vi "Stop Streaming.vi"(8 "error in (no error)":errorcluster, 11 "Camera in":refnum<class "Camera.lvclass">) -> (0 "error out":errorcluster, 3 "Camera":refnum<class "Camera.lvclass">)   [LabVIEW 2020, in "Camera.lvclass"]
doc: "Stop the camera streaming."
uses:
  Camera.lvclass
  Camera.lvclass/Camera.ctl
  bin/gindustrialcam_32-1.dll
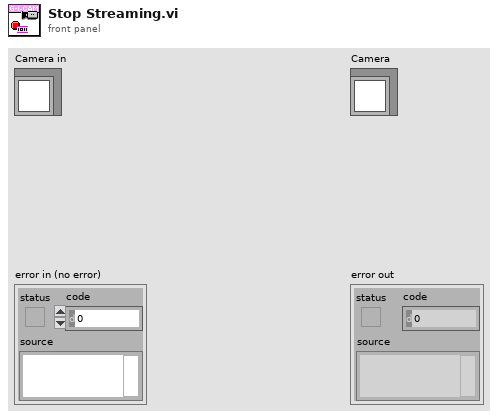
[diagram p1: front panel]
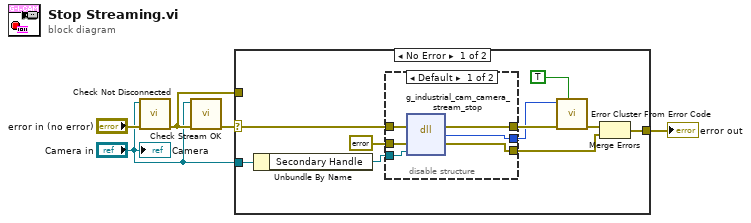
[diagram p0: block diagram]
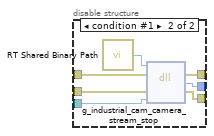
[diagram p2: hidden frame]
diagram:
  n1 = call "Check Not Disconnected.vi"("error in (no error)"="error in (no error)", "Camera in"="Camera in") -> ("error out"=w3:errorcluster)  [unwired: 9 in]
  n2 = call "Check Stream OK.vi"("error in (no error)"=w3, "Camera in"="Camera in") -> ("error out"=w1:errorcluster)  [unwired: 9 in]
  n3 = case shown="No Error" w1 {
    selector: w1 -> [w14 _]
    tunnel: [w15 w29] -> w4
    tunnel: w3 -> [_ w29]
    tunnel: "Camera in" -> [w7 _]
    frame No Error {
      n4 = Unbundle By Name(w7) -> ("Secondary Handle"=w6:refnum<data-value>)
      n5 = disable-structure shown="Default" {
        disable-tunnel: w14 -> [w21 w28]
        disable-tunnel: [w20 w27] -> w13
        disable-tunnel: [w19 w26] -> w12
        disable-tunnel: [w18 w25] -> w10
        disable-tunnel: errorcluster {"status"=FALSE, "code"=0, "source"=""} ("error constant") -> [w17 w24]
        disable-tunnel: w6 -> [w16 w23]
        frame condition #0 (active) {
          n6 = dll-call lib="C:/serenial/lib/g-industrial-camera/LabVIEW/g_industrial_cam/bin/gindustrialcam_*-1.*" fn="g_industrial_cam_camera_stream_stop"(error in=w21, "err"=w17, "cam_edvr"=w16) -> (error out=w20:errorcluster, "Mg_Error"=w19:i32, "err"=w18:errorcluster)  [unwired: 3 in, 1 out]
        }
        frame condition #1 {
          n7 = call "RT Shared Binary Path.vi"() -> ("Path"=w22:path)
          n8 = dll-call lib="C:/serenial/lib/g-industrial-camera/LabVIEW/g_industrial_cam/bin/gindustrialcam_*-1.*" fn="g_industrial_cam_camera_stream_stop"(path in=w22, error in=w28, "err"=w24, "cam_edvr"=w23) -> (error out=w27:errorcluster, "Mg_Error"=w26:i32, "err"=w25:errorcluster)  [unwired: 2 in, 1 out]
        }
      }
      n9 = call <vilib>:"Error Cluster From Error Code.vi"("show call chain? (False)"=TRUE, "error in (no error)"=w13, "error code (0)"=w12) -> ("error out"=w11:errorcluster)  [unwired: 6 in]
      n10 = Merge Errors(w11, w10) -> (w15:errorcluster)
    }
    frame Error {
    }
  }
  "error out" <- w4
  "Camera" <- "Camera in"
